vi "GetEvents.vi"(0 "SystemEvents.lvclass in":refnum<class "SystemEvents.lvclass">, 5 "error in (no error)":errorcluster) -> (14 "SystemEvents.lvclass out":refnum<class "SystemEvents.lvclass">, 16 "Events":T1, 19 "error out":errorcluster)   [LabVIEW 2017, in "SystemEvents.lvclass"]
doc: "Returns the Events attribute."
uses:
  SystemEvents.lvclass
  SystemEventData/SystemEventsType.ctl
  SystemEvents.lvclass/SystemEvents.ctl
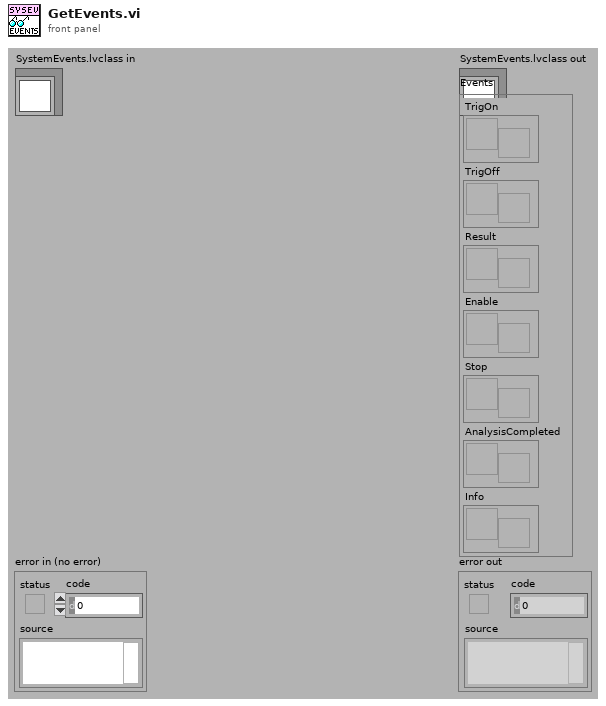
[diagram p1: front panel]
types:
  T1 = typedef "SystemEventsType.ctl" = cluster{"TrigOn":refnum<user-event>, "TrigOff":refnum<user-event>, "Result":refnum<user-event>, "Enable":refnum<user-event>, "Stop":refnum<user-event>, "AnalysisCompleted":refnum<user-event>, "Info":refnum<user-event>}
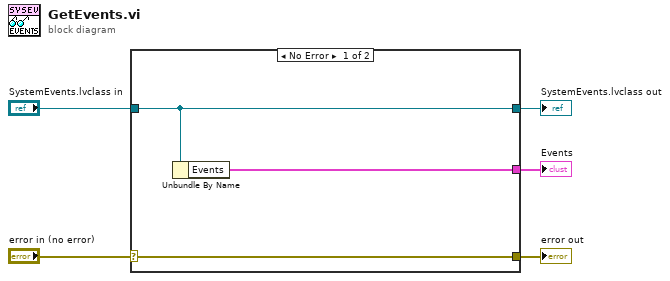
[diagram p0: block diagram]
diagram:
  n1 = case shown="No Error" "error in (no error)" {
    selector: "error in (no error)" -> [w8 w9]
    tunnel: [w8 w9] -> w4
    tunnel: [w7 w10] -> w2
    tunnel: "SystemEvents.lvclass in" -> [w7 w10]
    tunnel: [w6 _] -> w1
    frame No Error {
      n2 = Unbundle By Name(w7) -> ("Events"=w6:T1)
    }
    frame Error {
    }
  }
  "error out" <- w4
  "SystemEvents.lvclass out" <- w2
  "Events" <- w1
